vi "main.vi"() -> ()   [LabVIEW 2016]
uses:
  MyBaseActor/MyBaseActor/MyBaseActor.lvclass
  F:/Program Files (x86)/National Instruments/LabVIEW 2016/vi.lib/ActorFramework/Actor/Actor.lvclass
  MyBaseActor/MyBaseActor Messages/RequestStatus Msg/RequestStatus Msg.lvclass
  F:/Program Files (x86)/National Instruments/LabVIEW 2016/vi.lib/ActorFramework/Reply Msg/Reply Msg.lvclass
  <vilib>/ActorFramework/Reply Msg/Reply Msg.lvclass/Reply Msg.ctl
  <vilib>/ActorFramework/Message Enqueuer/Message Enqueuer.lvclass/Message Enqueuer.ctl
  <vilib>/ActorFramework/Message Enqueuer/Enqueue.vi
  <vilib>/ActorFramework/Reply Msg/Reply Msg.lvclass
  F:/Program Files (x86)/National Instruments/LabVIEW 2016/vi.lib/ActorFramework/Message/Message.lvclass
  <vilib>/ActorFramework/Stop Msg/Stop Msg.lvclass
  <vilib>/ActorFramework/Message Priority Queue/Priority Enqueue.vi
  <vilib>/ActorFramework/Actor/Actor.lvclass
panel:
  in  "Data":i32=1
  out "Reply (Data * 10)":i32
  # "1. Lauch \"MyBaseActor\"\n2. Request and return \"Status\" (blocking)\n3. Stop Actor\n4. Exit VI"
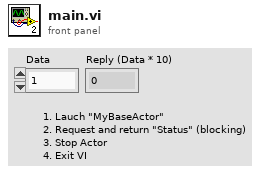
[diagram p1: front panel]
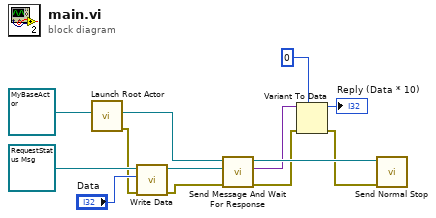
[diagram p0: block diagram]
diagram:
  n1 = call <vilib>:"Launch Root Actor.vi"("Actor"=refnum<class "MyBaseActor.lvclass"> refnum ("MyBaseActor.lvlib:MyBaseActor.lvclass")) -> ("error out"=w1:errorcluster, "Actor's Enqueuer"=w8:refnum<class "Message Enqueuer.lvclass">)  [unwired: 9 in]
  n2 = call-dynamic "Write Data.vi"("error in (no error)"=w1, "Data"="Data", "RequestStatus Msg in"=refnum<class "RequestStatus Msg.lvclass"> refnum ("MyBaseActor.lvlib:RequestStatus Msg.lvclass")) -> ("error out"=w10:errorcluster, "RequestStatus Msg out"=w11:refnum<class "RequestStatus Msg.lvclass">)  [unwired: 7 in]
  n3 = call <vilib>:"Send Message And Wait For Response.vi"("error in (no error)"=w10, "Original Message"=w11, "Message Enqueuer in"=w8) -> ("error out"=w3:errorcluster, "Reply"=w6:variant, "Message Enqueuer out"=w7:refnum<class "Message Enqueuer.lvclass">)  [unwired: 5 in, 1 out]
  n4 = Variant To Data(error in=w3, type=0 ("x*y"), Variant=w6) -> (data=→"Reply (Data * 10)":i32, error out=w2:errorcluster)
  n5 = call <vilib>:"Send Normal Stop.vi"("error in (no error)"=w2, "Message Enqueuer"=w7) -> ()  [unwired: 9 in, 1 out]
